vi "AddEventLog.vi"(8 "error in (no error)":errorcluster, 11 "Event":string) -> (0 "error out":errorcluster)   [LabVIEW 2023]
panel:
  in  "LogFile":path=path "C:/Users/Public/Documents/TVC Logs/errors.log"
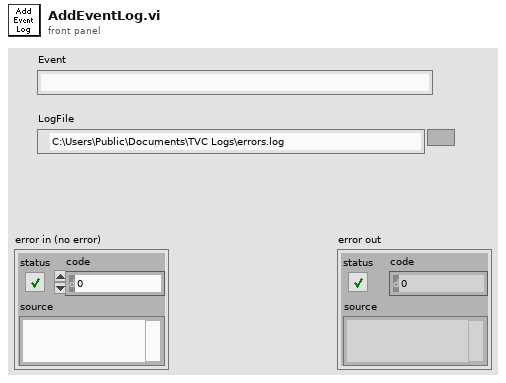
[diagram p1: front panel]
types:
  T1 = enum16{"open", "replace", "create", "open or create", "replace or create", "replace or create with confirmation"}
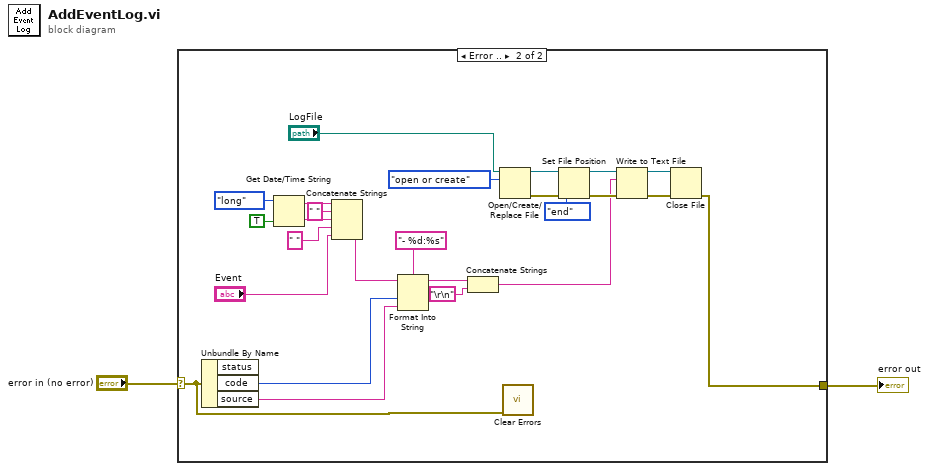
[diagram p0: block diagram]
diagram:
  n1 = case shown="Error .." "error in (no error)" {
    selector: "error in (no error)" -> [w3 w7]
    tunnel: [w3 w6] -> w1
    frame No Error {
    }
    frame Error {
      n2 = Unbundle By Name(w7) -> ("code"=w19:i32, "source"=w18:string)  [unwired: 1 out]
      n3 = Get Date/Time String(date format (0)=enum16{"short", "long", "abbreviated"}."long", want seconds? (F)=TRUE) -> (date string=w26:string, time string=w23:string)  [unwired: 1 in]
      n4 = Concatenate Strings(w26, " " ("string"), w23, " " ("string"), "Event") -> (w21:string)
      n5 = Format Into String(format string="- %d:%s", initial string=w21, w19, w18) -> (resulting string=w10:string)  [unwired: 1 in, 1 out]
      n6 = Concatenate Strings(w10, "\r\n") -> (w5:string)
      n7 = Open/Create/Replace File(file path (use dialog)="LogFile", operation (0:open)=T1."open or create") -> (refnum out=w14:refnum<file>, error out=w15:errorcluster)  [unwired: 4 in, 1 out]
      n8 = call <vilib>:"Clear Errors.vi"("error in (no error)"=w7) -> ()  [unwired: 5 in, 2 out]
      n9 = Set File Position(refnum=w14, from (0:start)=enum16{"start", "end", "current"}."end", error in=w15) -> (refnum out=w11:refnum<file>, error out=w12:errorcluster)  [unwired: 1 in]
      n10 = Write to Text File(file (use dialog)=w11, text=w5, error in=w12) -> (refnum out=w8:refnum<file>, error out=w9:errorcluster)  [unwired: 1 in, 1 out]
      n11 = Close File(refnum=w8, error in=w9) -> (error out=w6:errorcluster)  [unwired: 1 out]
    }
  }
  "error out" <- w1
